vi "uTTA_Read_File_UI.vi"(4 "error in":errorcluster, 6 "Externally Called":bool, 7 "VISA resource name":refnum<visa-resource-name>) -> (0 "error out":errorcluster)   [LabVIEW 2021]
panel:
  out "Connected":bool
  in  "Delete":bool
  out "Last Line":string
  in  "EXIT":bool
  in  "File":u16(ring)
  in  "Connect":bool
  in  "Read":bool
  out "RunTime":dbl format="%ds"
  out "Read took":i32 format="%.0fms"
  out "Timeout Expanded":bool
  out "Received":string
  out "error RT":errorcluster
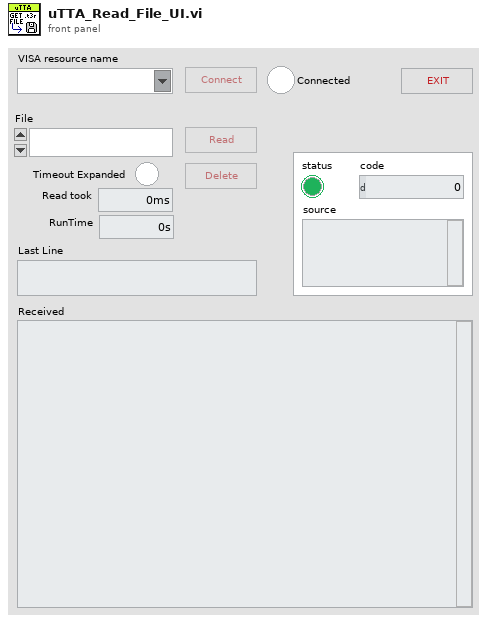
[diagram p1: front panel]
types:
  T1 = enum8{"Enabled", "Disabled", "Disabled and Grayed Out"}
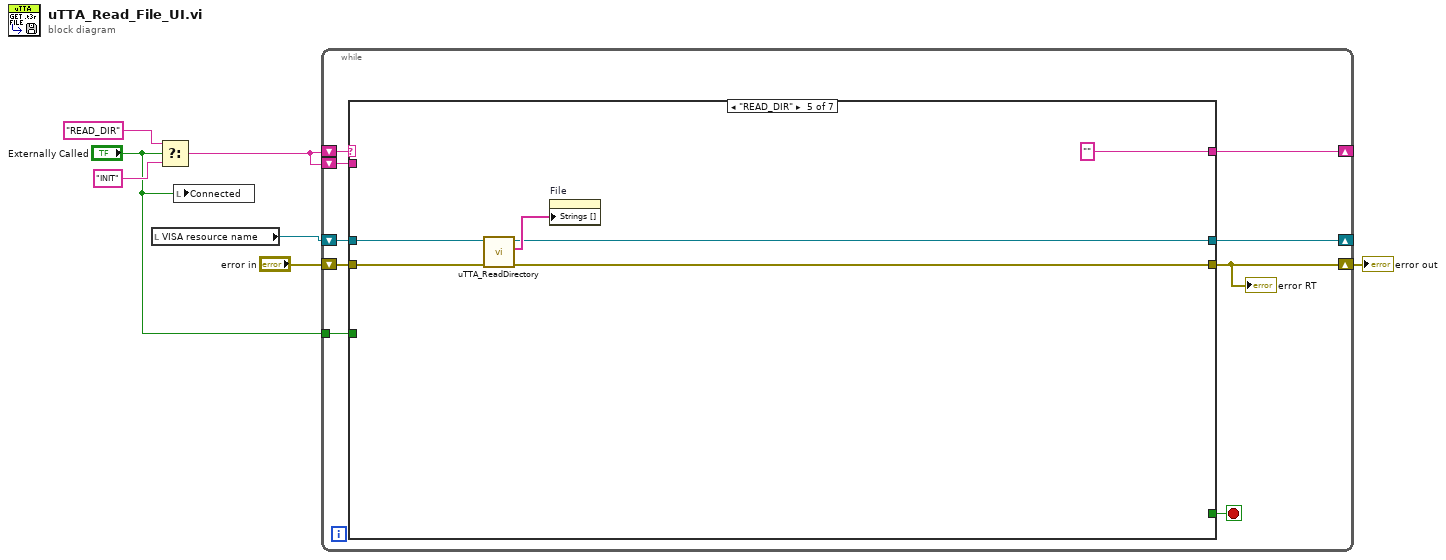
[diagram p0: block diagram]
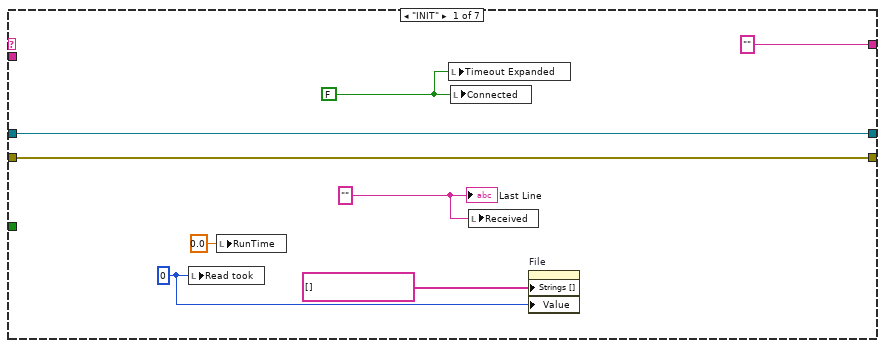
[diagram p2: hidden frame]
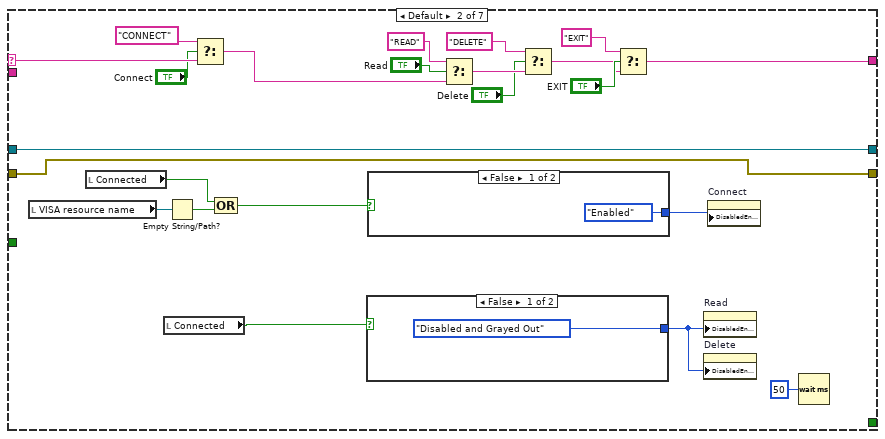
[diagram p3: hidden frame]
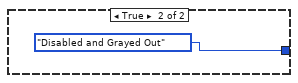
[diagram p4: hidden frame]
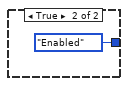
[diagram p5: hidden frame]
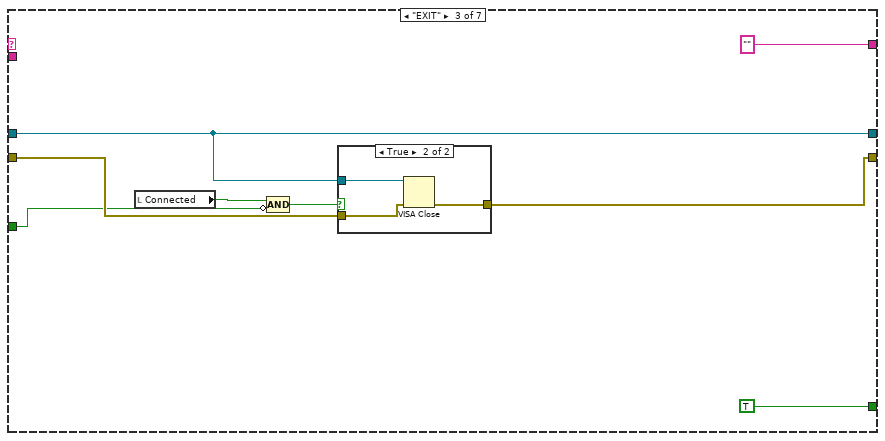
[diagram p6: hidden frame]
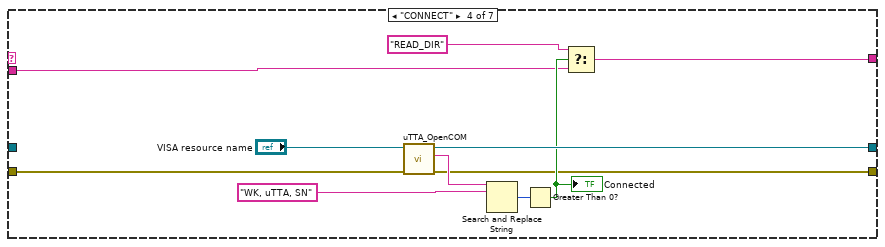
[diagram p8: hidden frame]
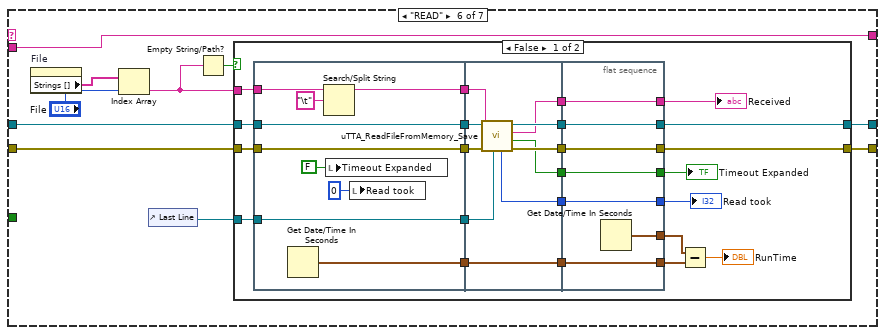
[diagram p9: hidden frame]
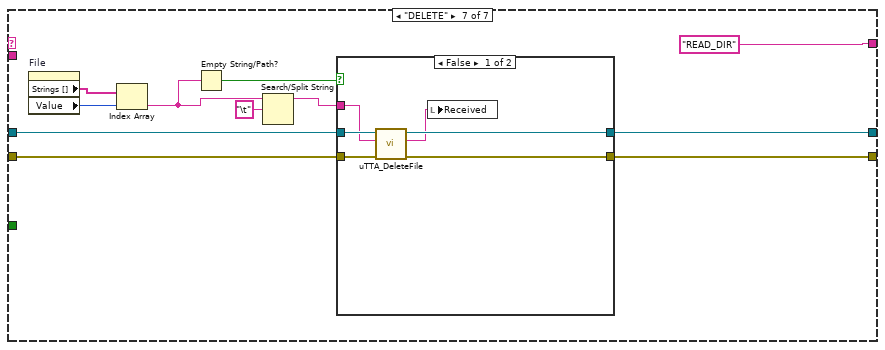
[diagram p11: hidden frame]
diagram:
  n1 = local read "VISA resource name"() -> (w1:refnum<visa-resource-name>)
  n2 = Select(t="READ_DIR", s="Externally Called", f="INIT" ("Filename")) -> (s? t:f=w4:string)
  n3 = local write "Connected"("Externally Called") -> ()
  n4 = while {
    shift-right: [w14] -> _
    shift-left: w4 -> [w15]
    shift-right: [w13] -> _
    shift-left: w1 -> [w12]
    shift-left: w4 -> [w11]
    shift-right: [w9] -> w6
    shift-left: "error in" -> [w10]
    tunnel: "Externally Called" -> [w8]
    stop <- w16 stop-if-true
    n5 = case shown="\"READ_DIR\"" w15 {
      selector: w15 -> [_ w42 _ _ _ _ _]
      tunnel: [_ _ TRUE ("EXIT") _ _ _ _] -> w16
      tunnel: ["" ("t") w30 "" ("t") w67 "" ("Filename") w83 "READ_DIR" ("t")] -> w14
      tunnel: [w20 w28 w58 w73 w78 w85 w147] -> w13
      tunnel: w12 -> [w20 w28 w58 _ w79 w84 w148]
      tunnel: w11 -> [_ _ _ w66 _ w83 _]
      tunnel: w10 -> [w17 w26 w56 w65 w76 w82 w146]
      tunnel: [w17 w26 w55 w64 w75 w81 w145] -> w9
      tunnel: w8 -> [_ _ w53 _ _ _ _]
      frame "INIT" {
        w19 = 0 ("Read took ms")
        w23 = "" ("Last Line")
        w18 = FALSE ("Connected")
        n6 = local write "Read took"(w19) -> ()
        n7 = local write "RunTime"(0.0 ("RunTime")) -> ()
        n8 = local write "Timeout Expanded"(w18) -> ()
        n9 = local write "Connected"(w18) -> ()
        n10 = local write "Received"(w23) -> ()
        n11 = property on="File" class="Ring (strict)"("Strings []"=string[] [], "Value"=w19) -> ()  [unwired: 2 in, 2 out]
        "Last Line" <- w23
      }
      frame Default {
        n12 = local read "VISA resource name"() -> (w45:refnum<visa-resource-name>)
        n13 = local read "Connected"() -> (w27:bool)
        n14 = local read "Connected"() -> (w25:bool)
        n15 = Empty String/Path?(string/path=w45) -> (empty?=w34:bool)
        n16 = Select(t="CONNECT", s="Connect", f=w42) -> (s? t:f=w41:string)
        n17 = Compound Arithmetic op=OR(w27, w34) -> (w33:bool)
        n18 = case shown="False" w25 {
          tunnel: [T1."Disabled and Grayed Out" ("Disabled") T1."Enabled" ("Disabled")] -> w35
          frame False {
          }
          frame True {
          }
        }
        n19 = case shown="False" w33 {
          tunnel: [T1."Enabled" ("Disabled") T1."Disabled and Grayed Out" ("Disabled")] -> w43
          frame False {
          }
          frame True {
          }
        }
        n20 = Select(t="READ" ("Filename"), s="Read", f=w41) -> (s? t:f=w38:string)
        n21 = Select(t="DELETE", s="Delete", f=w38) -> (s? t:f=w31:string)
        n22 = Select(t="EXIT", s="EXIT", f=w31) -> (s? t:f=w30:string)
        n23 = property on="Read" class="Bool"("DisabledEnum"=w35) -> ()  [unwired: 2 in, 2 out]
        n24 = property on="Delete" class="Bool"("DisabledEnum"=w35) -> ()  [unwired: 2 in, 2 out]
        n25 = property on="Connect" class="Bool"("DisabledEnum"=w43) -> ()  [unwired: 2 in, 2 out]
        n26 = Wait (ms)(milliseconds to wait=u32 50) -> ()  [unwired: 1 out]
      }
      frame "EXIT" {
        n27 = local read "Connected"() -> (w54:bool)
        n28 = Compound Arithmetic op=AND(w54, invert w53) -> (w52:bool)
        n29 = case shown="True" w52 {
          tunnel: w58 -> [_ w63]
          tunnel: w56 -> [w60 w62]
          tunnel: [w60 w61] -> w55
          frame False {
          }
          frame True {
            n30 = VISA Close(VISA resource name=w63, error in (no error)=w62) -> (error out=w61:errorcluster)
          }
        }
      }
      frame "CONNECT" {
        n31 = call "uTTA_OpenCOM.vi"("error in"=w65, "VISA in"="VISA resource name") -> ("error out"=w64:errorcluster, "Identity"=w71:string, "VISA out"=w73:refnum<visa-resource-name>)  [unwired: 7 in]
        n32 = Search and Replace String(input string=w71, search string="WK, uTTA, SN") -> (number of replacements=w72:i32)  [unwired: 6 in, 3 out]
        n33 = Greater Than 0?(x=w72) -> (x > 0?=w68:bool)
        "Connected" <- w68
        n34 = Select(t="READ_DIR", s=w68, f=w66) -> (s? t:f=w67:string)
      }
      frame "READ_DIR" {
        n35 = call "uTTA_ReadDirectory.vi"("error in"=w76, "VISA Refnum in"=w79) -> ("error out"=w75:errorcluster, "Files"=w80:string[], "VISA Refnum out"=w78:refnum<visa-resource-name>)  [unwired: 3 in]
        n36 = property on="File" class="Ring (strict)"("Strings []"=w80) -> ()  [unwired: 2 in, 2 out]
      }
      frame "READ" {
        n37 = property on="File" class="Ring (strict)"() -> ("Strings []"=w90:string[])  [unwired: 2 in, 2 out]
        n38 = Index Array(array=w90, index="File") -> (element=w87:string)
        n39 = control-ref of="Last Line"() -> (w86:refnum<vi>)
        n40 = Empty String/Path?(string/path=w87) -> (empty?=w88:bool)
        n41 = case shown="False" w88 {
          tunnel: w84 -> [w99 w141]
          tunnel: w87 -> [w98 _]
          tunnel: w86 -> [w97 _]
          tunnel: [w95 w141] -> w85
          tunnel: w82 -> [w94 w140]
          tunnel: [w92 w140] -> w81
          frame False {
            n42 = flat-sequence {
              tunnel: w98 -> [w116]
              tunnel: w99 -> [w122]
              tunnel: [w122] -> w113
              tunnel: [w121] -> w112
              tunnel: w97 -> [w120]
              tunnel: [w120] -> w96
              tunnel: w94 -> [w119]
              tunnel: [w119] -> w93
              tunnel: [w114] -> w91
              tunnel: w113 -> [w132]
              tunnel: [w131] -> w111
              tunnel: [w130] -> w110
              tunnel: [w128] -> w109
              tunnel: [w127] -> w108
              tunnel: [w126] -> w107
              tunnel: [w125] -> w106
              tunnel: w112 -> [w125]
              tunnel: w96 -> [w124]
              tunnel: w93 -> [w123]
              tunnel: w91 -> [w129]
              tunnel: [w135] -> w103
              tunnel: [w136] -> w104
              tunnel: [w137] -> w105
              tunnel: [w138] -> w95
              tunnel: [w139] -> w92
              tunnel: w111 -> [w139]
              tunnel: w110 -> [w138]
              tunnel: w109 -> [w137]
              tunnel: w108 -> [w136]
              tunnel: w107 -> [w135]
              tunnel: [w134] -> w102
              tunnel: w106 -> [w134]
              tunnel: [w133] -> w101
              frame #0 {
                n43 = Get Date/Time In Seconds() -> (seconds since 1Jan1904=w121:timestamp)
                n44 = Search/Split String(string=w116, search string/char (-)="\t") -> (substring before match=w114:string)  [unwired: 1 in, 2 out]
                n45 = local write "Timeout Expanded"(FALSE ("Timeout Expanded")) -> ()
                n46 = local write "Read took"(0 ("Read took")) -> ()
              }
              frame #1 {
                n47 = call "uTTA_ReadFileFromMemory_Save.vi"("Last Line"=w124, "error in"=w123, "Filename"=w129, "VISA Refnum in"=w132) -> ("error out"=w131:errorcluster, "Timeout Expanded"=w127:bool, "Received"=w128:string, "VISA Refnum out"=w130:refnum<visa-resource-name>, "Read took ms"=w126:i32)  [unwired: 3 in]
              }
              frame #2 {
                n48 = Get Date/Time In Seconds() -> (seconds since 1Jan1904=w133:timestamp)
              }
            }
            n49 = Subtract(x=w101, y=w102) -> (x-y=→"RunTime":dbl)
            "Received" <- w105
            "Timeout Expanded" <- w104
            "Read took" <- w103
          }
          frame True {
          }
        }
      }
      frame "DELETE" {
        n50 = property on="File" class="Ring (strict)"() -> ("Strings []"=w149:string[], "Value"=w151:u16)  [unwired: 2 in, 2 out]
        n51 = Index Array(array=w149, index=w151) -> (element=w143:string)
        n52 = Empty String/Path?(string/path=w143) -> (empty?=w150:bool)
        n53 = Search/Split String(string=w143, search string/char (-)="\t") -> (substring before match=w142:string)  [unwired: 1 in, 2 out]
        n54 = case shown="False" w150 {
          tunnel: w142 -> [w157 _]
          tunnel: w148 -> [w158 w160]
          tunnel: [w156 w160] -> w147
          tunnel: w146 -> [w154 w159]
          tunnel: [w153 w159] -> w145
          frame False {
            n55 = call "uTTA_DeleteFile.vi"("error in"=w154, "Directory Name"=w157, "VISA Refnum in"=w158) -> ("error out"=w153:errorcluster, "Received"=w155:string, "VISA Refnum out"=w156:refnum<visa-resource-name>)  [unwired: 2 in]
            n56 = local write "Received"(w155) -> ()
          }
          frame True {
          }
        }
      }
    }
    "error RT" <- w9
  }
  "error out" <- w6
